vi "DPO_7K_Communication_Settings.vi"(8 "Error In":errorcluster, 11 "VISA resource name in":refnum<visa-resource-name>) -> (0 "error out":errorcluster, 3 "VISA resource name out":refnum<visa-resource-name>)   [LabVIEW 2020]
doc: "Establishes communication with the instrument and optionally performs an instrument identification query or an instrument reset. This VI also places the instrument in a default state needed for other instrument driver operations.\nRun this VI before running other instrument driver VIs for the instrument. You generally need to run the Initialize VI only once, at the beginning of an application."
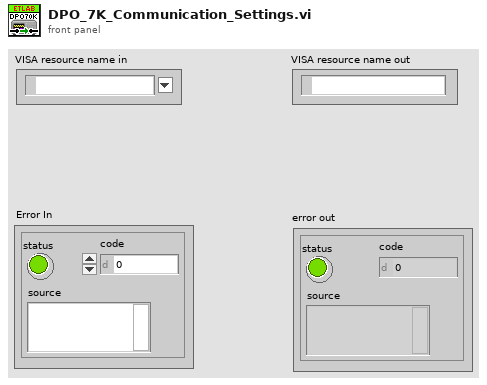
[diagram p1: front panel]
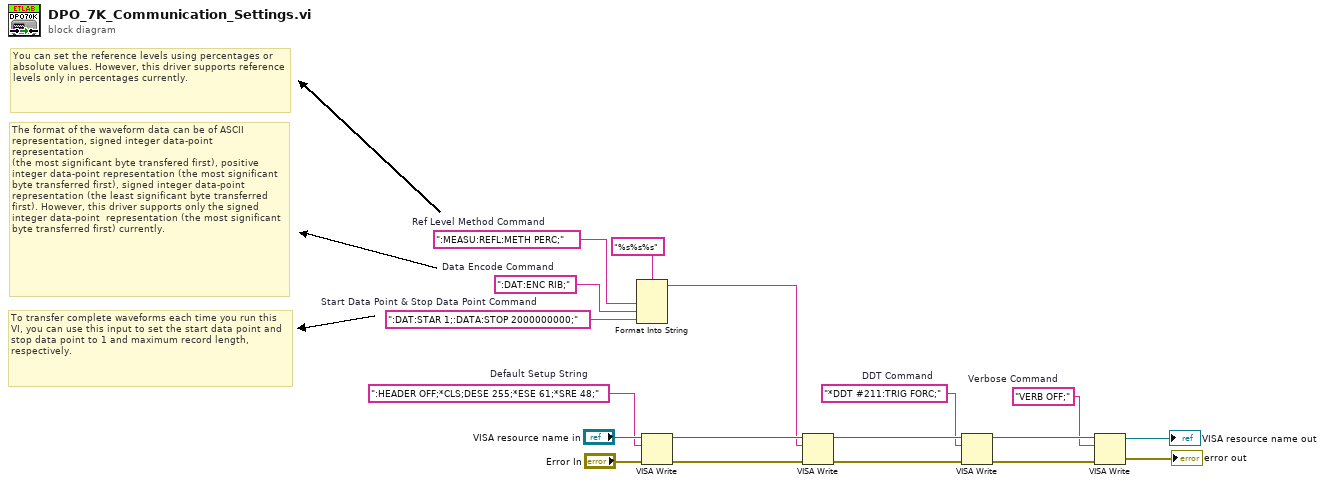
[diagram p0: block diagram]
diagram:
  w3 = ":DAT:STAR 1;:DATA:STOP 2000000000;"  # Start Data Point & Stop Data Point Command
  w4 = ":DAT:ENC RIB;"  # Data Encode Command
  w5 = ":HEADER OFF;*CLS;DESE 255;*ESE 61;*SRE 48;"  # Default Setup String
  w6 = "VERB OFF;"  # Verbose Command
  w9 = "*DDT #211:TRIG FORC;"  # DDT Command
  w16 = ":MEASU:REFL:METH PERC;"  # Ref Level Method Command
  # "To transfer complete waveforms each time you run this VI, you can use this input to set the start data point and stop data point to 1 and maximum record length, respectively."
  # "The format of the waveform data can be of ASCII\nrepresentation, signed integer data-point representation \n(the most significant byte transfered first), positive \ninteger data-point representation (the most significant \nbyte transferred first), signed integer data-point \nrepresentation (the least significant byte transferred first). However, this driver supports only the signed integer data-point  representation (the most significant byte transferred first) currently."
  # "You can set the reference levels using percentages or absolute values. However, this driver supports reference levels only in percentages currently."
  n1 = Format Into String(format string="%s%s%s", w16, w4, w3) -> (resulting string=w13:string)  [unwired: 2 in, 1 out]
  n2 = VISA Write(VISA resource name="VISA resource name in", write buffer=w5, error in (no error)="Error In") -> (VISA resource name out=w15:refnum<visa-resource-name>, error out=w14:errorcluster)  [unwired: 1 out]
  n3 = VISA Write(VISA resource name=w15, write buffer=w13, error in (no error)=w14) -> (VISA resource name out=w11:refnum<visa-resource-name>, error out=w10:errorcluster)  [unwired: 1 out]
  n4 = VISA Write(VISA resource name=w11, write buffer=w9, error in (no error)=w10) -> (VISA resource name out=w8:refnum<visa-resource-name>, error out=w7:errorcluster)  [unwired: 1 out]
  n5 = VISA Write(VISA resource name=w8, write buffer=w6, error in (no error)=w7) -> (VISA resource name out=→"VISA resource name out":refnum<visa-resource-name>, error out=→"error out":errorcluster)  [unwired: 1 out]
